vi "getDt.vi"() -> (0 "dt(s)":dbl)   [LabVIEW 2014]
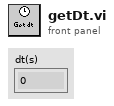
[diagram p1: front panel]
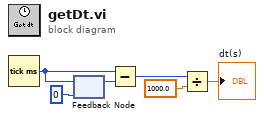
[diagram p0: block diagram]
diagram:
  n1 = Tick Count (ms)() -> (millisecond timer value=w4:u32)
  n2 = feedback-in #1(w4) -> ()
  n3 = feedback #1(u32 0 ("millisecond timer value")) -> (w5:u32)
  n4 = Subtract(x=w4, y=w5) -> (x-y=w1:u32)
  n5 = Divide(x=w1, y=1000.0) -> (x/y=→"dt(s)":dbl)
